vi "DROPBEAR_Model_Updating_Store_Statisitics.vi"(8 "error in (no error)":errorcluster, 11 "DROPBEAR_Model_Updating in":refnum<class "DROPBEAR_Model_Updating.lvclass">) -> (0 "error out":errorcluster, 3 "DROPBEAR_Model_Updating out":refnum<class "DROPBEAR_Model_Updating.lvclass">)   [LabVIEW 2021, in "DROPBEAR_Model_Updating.lvclass"]
uses:
  DROPBEAR_Model_Updating.lvclass
  DROPBEAR_Model_Updating.lvclass/DROPBEAR_Model_Updating.ctl
  Online_Statistic/Online_Statistic.lvclass/Online_Statistic.ctl
  Read Record Statistics.vi
  Write Time Cycle End.vi
  Read Distributional Statistics.vi
  Read Time Flags.vi
  Online_Statistic/Read Cumulative_mean.vi
  Write Distributional Statistics.vi
  Read Online Cycle Time Cost.vi
  Read Time Cycle Start.vi
  Read Time Cycle End.vi
  Write Online Cycle Time Cost.vi
  Read Record Moving Window Data.vi
  Read Record Time Series Data.vi
  Read Pinned State KF.vi
  Read Record Online Error Metrics .vi
  Read Online_SNR_Frequency.vi
  Read Online_SNR_Position_Meters.vi
  Read Online_TRAC_Frequency.vi
  Read Online_TRAC_Meters.vi
  Read Model_Error_Frequency.vi
  Read Model_Error_Meters.vi
  Write Online_SNR_Frequency.vi
  Write Online_SNR_Position_Meters.vi
  Write Online_TRAC_Frequency.vi
  Write Online_TRAC_Meters.vi
  Write Model_Error_Frequency.vi
  Write Model_Error_Meters.vi
  Read Store Statistics Time Cost.vi
  Write Time Store Satistics.vi
  Write Store Statistics Time Cost.vi
  Online_Statistic/Online_Statistic.lvclass
  Moving_Statistic/Moving_Statistic.lvclass
  Data_Array/Data_Array.lvclass
  Kalman_Filter/Kalman_Filter.lvclass
  Online_SNR/Online_SNR.lvclass
  Online_TRAC/Online_TRAC.lvclass
  MOCKBEAR/MOCKBEAR.lvclass
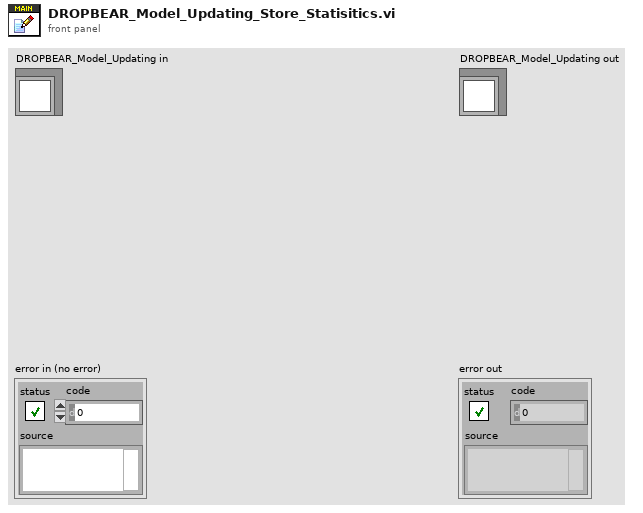
[diagram p1: front panel]
types:
  T1 = cluster{"Data Acquistion Time Cost":refnum<class "Online_Statistic.lvclass">, "FFT Time Cost":refnum<class "Online_Statistic.lvclass">, "Frequency Tracking Time Cost":refnum<class "Online_Statistic.lvclass">, "Sample Location Time Cost":refnum<class "Online_Statistic.lvclass">, "FEA Time Cost":refnum<class "Online_Statistic.lvclass">, "State Tracking Time Cost":refnum<class "Online_Statistic.lvclass">, "Online Cycle Time Cost":refnum<class "Online_Statistic.lvclass">, "Store Statistics Time Cost":refnum<class "Online_Statistic.lvclass">}
  T2 = cluster{"Time Cycle Start":u32, "Time Data Acquire":u32, "Time FFT":u32, "Time KF FFT":u32, "Time Sample":u32, "Time FEA":u32, "Time KF FEA":u32, "Time Cycle End":u32, "Time Store Satistics":u32}
  T3 = cluster{"Displacement Measured Meters":refnum<class "Moving_Statistic.lvclass">, "Displacement Estimate Meters":refnum<class "Moving_Statistic.lvclass">, "Frequency Measured":refnum<class "Moving_Statistic.lvclass">, "Frequency at Estimate":refnum<class "Moving_Statistic.lvclass">}
  T4 = cluster{"Position Measured Meters":dbl, "Position Measured Nodal":i32, "Position Estimated Meters":dbl, "Position Estimated Nodal":i32, "Frequency Estimated KF":dbl, "Frequency Measured FFT":dbl, "Position Estimated Meters KF":dbl, "Position Estimated Nodal KF":i32, "Mean Cycle time":dbl, "Frequency True Position":dbl}
  T5 = cluster{"Modeling Parameters input controls":cluster{"beam_length":dbl, "youngs_modulus":dbl, "torsion_spring":dbl, "beam_height":dbl, "beam_width":dbl, "beam_density":dbl, "number_of_FEA_nodes":i32, "accelerometer_mass":dbl}, "Mockbear input controls":cluster{"Dataset":string, "Resample Method":enum16{"Recorded", "Auto Resample", "Custom Resample"}}, "Simulation Parameters input controls":cluster{"Eigensolver ":enum16{"LabVIEW Cholesky", "LabVIEW General", "LabVIEW Inverse", "LEMP"}, "Models Forcasted":i32, "Max Roller Velocity":dbl, "Max Roller Position Percent":dbl, "Min Roller Position Percent":dbl}, "Program Controls":cluster{"Frequency KF":bool, "Pinned State KF":bool, "FFT Bounding":bool, "Filter Constants Frequency":cluster{"Measurement Variance":dbl, "State Variance":dbl, "Threshold":dbl}, "Filter Constants Position":cluster{"Measurement Variance":dbl, "State Variance":dbl, "Threshold":dbl}, "Moving Window Size":i32, "Time Series buffer":dbl, "Record Time Series Data":bool, "Record Moving Window Data":bool, "Record Online Error Metrics ":bool, "Record Statistics":bool}}
  T6 = cluster{"Frequency KF":bool, "Pinned State KF":bool, "FFT Bounding":bool, "Filter Constants Frequency":cluster{"Measurement Variance":dbl, "State Variance":dbl, "Threshold":dbl}, "Filter Constants Position":cluster{"Measurement Variance":dbl, "State Variance":dbl, "Threshold":dbl}, "Moving Window Size":i32, "Time Series buffer":dbl, "Record Time Series Data":bool, "Record Moving Window Data":bool, "Record Online Error Metrics ":bool, "Record Statistics":bool}
  T7 = cluster{"Displacement Measured Nodal ":refnum<class "Data_Array.lvclass">, "Displacement Measured Meters":refnum<class "Data_Array.lvclass">, "Displacement Estimate Nodal":refnum<class "Data_Array.lvclass">, "Displacement Estimate Meters":refnum<class "Data_Array.lvclass">, "Frequency Measured":refnum<class "Data_Array.lvclass">, "Frequency at Estimate":refnum<class "Data_Array.lvclass">}
  T8 = cluster{"Frequency State":refnum<class "Kalman_Filter.lvclass">, "Rolling Condition State":refnum<class "Kalman_Filter.lvclass">, "Frequency State":dbl, "Pinned Condition State":dbl}
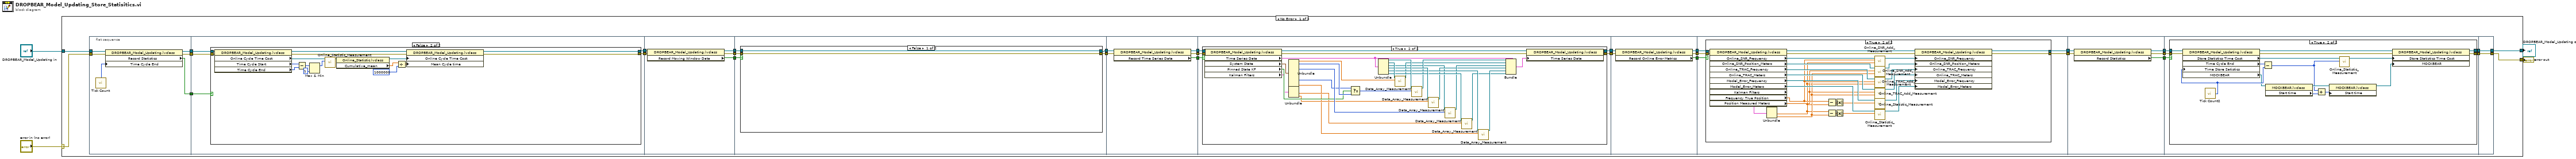
[diagram p0: block diagram]
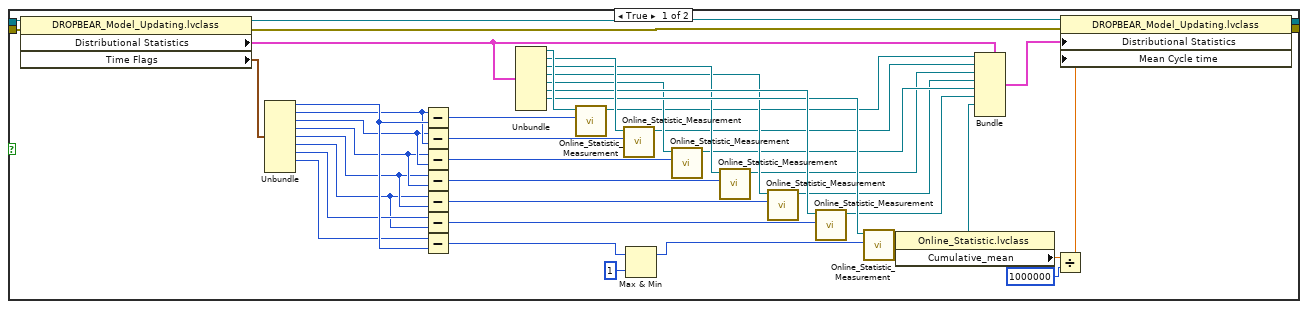
[diagram p2: hidden frame]
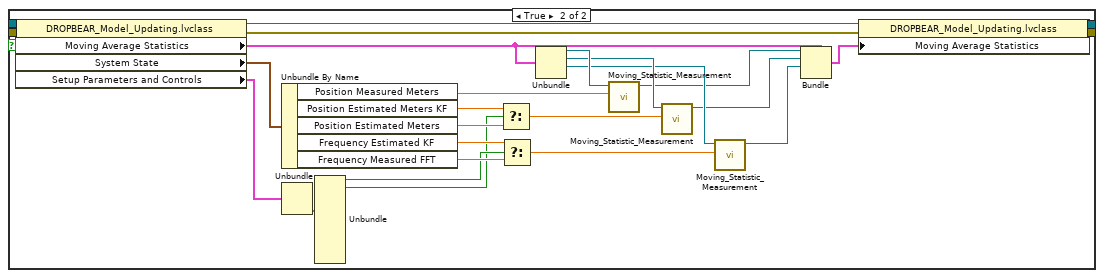
[diagram p3: hidden frame]
diagram:
  n1 = case shown="No Error" "error in (no error)" {
    selector: "error in (no error)" -> [w31 w257]
    tunnel: [w12 w257] -> w3
    tunnel: [w32 w256] -> w1
    tunnel: "DROPBEAR_Model_Updating in" -> [w33 w256]
    frame No Error {
      n2 = flat-sequence {
        tunnel: w31 -> [w38]
        tunnel: w33 -> [w39]
        tunnel: [w37] -> w22
        tunnel: [w36] -> w21
        tunnel: [w35] -> w18
        tunnel: [w44] -> w24
        tunnel: [w43] -> w26
        tunnel: w21 -> [w41]
        tunnel: w22 -> [w42]
        tunnel: w18 -> [w40]
        tunnel: w26 -> [w109]
        tunnel: [w107] -> w25
        tunnel: w24 -> [w110]
        tunnel: [w108] -> w23
        tunnel: [w106] -> w17
        tunnel: [w115] -> w28
        tunnel: [w114] -> w30
        tunnel: w25 -> [w112]
        tunnel: w23 -> [w113]
        tunnel: w17 -> [w111]
        tunnel: w30 -> [w147]
        tunnel: [w145] -> w29
        tunnel: w28 -> [w148]
        tunnel: [w146] -> w27
        tunnel: [w144] -> w16
        tunnel: w29 -> [w150]
        tunnel: w27 -> [w151]
        tunnel: [w153] -> w20
        tunnel: [w152] -> w19
        tunnel: w16 -> [w149]
        tunnel: w20 -> [w191]
        tunnel: w19 -> [w190]
        tunnel: [w189] -> w15
        tunnel: [w188] -> w14
        tunnel: [w187] -> w13
        tunnel: w15 -> [w196]
        tunnel: w14 -> [w195]
        tunnel: w13 -> [w192]
        tunnel: [w194] -> w9
        tunnel: [w193] -> w7
        tunnel: w9 -> [w230]
        tunnel: [w228] -> w8
        tunnel: w7 -> [w229]
        tunnel: [w227] -> w6
        tunnel: [w226] -> w5
        tunnel: w8 -> [w235]
        tunnel: w6 -> [w234]
        tunnel: [w233] -> w11
        tunnel: [w232] -> w10
        tunnel: w5 -> [w231]
        tunnel: [w254] -> w12
        tunnel: [w255] -> w32
        tunnel: w11 -> [w255]
        tunnel: w10 -> [w254]
        frame #0 {
          n3 = call "Tick Count"() -> ("Tick Count(uSec)"=w34:u32)
          n4 = property class="DROPBEAR_Model_Updating.lvclass"(reference=w39, error in=w38, "Time Cycle End"=w34) -> (reference out=w37:refnum<class "DROPBEAR_Model_Updating.lvclass">, error out=w36:errorcluster, "Record Statistics"=w35:bool)
        }
        frame #1 {
          n5 = case shown="False" w40 {
            tunnel: [w66 w104] -> w44
            tunnel: [w64 w102] -> w43
            tunnel: w42 -> [w61 w99]
            tunnel: w41 -> [w51 w98]
            frame True {
              n6 = property class="DROPBEAR_Model_Updating.lvclass"(reference=w61, error in=w51) -> (reference out=w68:refnum<class "DROPBEAR_Model_Updating.lvclass">, error out=w65:errorcluster, "Distributional Statistics"=w75:T1, "Time Flags"=w60:T2)
              n7 = Unbundle(w60) -> ("Time Cycle Start"=w59:u32, "Time Data Acquire"=w56:u32, "Time FFT"=w55:u32, "Time KF FFT"=w54:u32, "Time Sample"=w53:u32, "Time FEA"=w52:u32, "Time KF FEA"=w58:u32, "Time Cycle End"=w57:u32)  [unwired: 1 out]
              n8 = Subtract(x=w56, y=w59) -> (x-y=w88:u32)
              n9 = Subtract(x=w55, y=w56) -> (x-y=w87:u32)
              n10 = Subtract(x=w54, y=w55) -> (x-y=w86:u32)
              n11 = Subtract(x=w53, y=w54) -> (x-y=w85:u32)
              n12 = Subtract(x=w52, y=w53) -> (x-y=w84:u32)
              n13 = Subtract(x=w58, y=w52) -> (x-y=w83:u32)
              n14 = Subtract(x=w57, y=w59) -> (x-y=w47:u32)
              n15 = Unbundle(w75) -> ("Data Acquistion Time Cost"=w82:refnum<class "Online_Statistic.lvclass">, "FFT Time Cost"=w81:refnum<class "Online_Statistic.lvclass">, "Frequency Tracking Time Cost"=w77:refnum<class "Online_Statistic.lvclass">, "Sample Location Time Cost"=w76:refnum<class "Online_Statistic.lvclass">, "FEA Time Cost"=w78:refnum<class "Online_Statistic.lvclass">, "State Tracking Time Cost"=w80:refnum<class "Online_Statistic.lvclass">, "Online Cycle Time Cost"=w79:refnum<class "Online_Statistic.lvclass">)  [unwired: 1 out]
              n16 = call-dynamic "Online_Statistic_Measurement.vi"("New_Measurement"=w88, "Online_Statistic in"=w82) -> ("Online_Statistic out"=w74:refnum<class "Online_Statistic.lvclass">)  [unwired: 8 in, 1 out]
              n17 = call-dynamic "Online_Statistic_Measurement.vi"("New_Measurement"=w87, "Online_Statistic in"=w81) -> ("Online_Statistic out"=w73:refnum<class "Online_Statistic.lvclass">)  [unwired: 8 in, 1 out]
              n18 = Max & Min(x=w47, y=u32 1) -> (max(x,y)=w46:u32)  [unwired: 1 out]
              n19 = call-dynamic "Online_Statistic_Measurement.vi"("New_Measurement"=w86, "Online_Statistic in"=w78) -> ("Online_Statistic out"=w72:refnum<class "Online_Statistic.lvclass">)  [unwired: 8 in, 1 out]
              n20 = call-dynamic "Online_Statistic_Measurement.vi"("New_Measurement"=w85, "Online_Statistic in"=w77) -> ("Online_Statistic out"=w71:refnum<class "Online_Statistic.lvclass">)  [unwired: 8 in, 1 out]
              n21 = call-dynamic "Online_Statistic_Measurement.vi"("New_Measurement"=w84, "Online_Statistic in"=w76) -> ("Online_Statistic out"=w70:refnum<class "Online_Statistic.lvclass">)  [unwired: 8 in, 1 out]
              n22 = call-dynamic "Online_Statistic_Measurement.vi"("New_Measurement"=w83, "Online_Statistic in"=w80) -> ("Online_Statistic out"=w69:refnum<class "Online_Statistic.lvclass">)  [unwired: 8 in, 1 out]
              n23 = call-dynamic "Online_Statistic_Measurement.vi"("New_Measurement"=w46, "Online_Statistic in"=w79) -> ("Online_Statistic out"=w50:refnum<class "Online_Statistic.lvclass">)  [unwired: 8 in, 1 out]
              n24 = property class="Online_Statistic.lvclass"(reference=w50) -> (reference out=w49:refnum<class "Online_Statistic.lvclass">, "Cumulative_mean"=w48:dbl)  [unwired: 1 in, 1 out]
              n25 = Bundle(cluster=w75, "Data Acquistion Time Cost"=w74, "FFT Time Cost"=w73, "Frequency Tracking Time Cost"=w71, "Sample Location Time Cost"=w70, "FEA Time Cost"=w72, "State Tracking Time Cost"=w69, "Online Cycle Time Cost"=w49) -> (w67:T1)  [unwired: 1 in]
              n26 = Divide(x=w48, y=u32 1000000) -> (x/y=w62:dbl)
              n27 = property class="DROPBEAR_Model_Updating.lvclass"(reference=w68, error in=w65, "Distributional Statistics"=w67, "Mean Cycle time"=w62) -> (reference out=w66:refnum<class "DROPBEAR_Model_Updating.lvclass">, error out=w64:errorcluster)
            }
            frame False {
              n28 = property class="DROPBEAR_Model_Updating.lvclass"(reference=w99, error in=w98) -> (reference out=w105:refnum<class "DROPBEAR_Model_Updating.lvclass">, error out=w103:errorcluster, "Online Cycle Time Cost"=w95:refnum<class "Online_Statistic.lvclass">, "Time Cycle Start"=w93:u32, "Time Cycle End"=w92:u32)
              n29 = Subtract(x=w93, y=w92) -> (x-y=w90:u32)
              n30 = Max & Min(x=w90, y=1) -> (max(x,y)=w89:u32)  [unwired: 1 out]
              n31 = call-dynamic "Online_Statistic_Measurement.vi"("New_Measurement"=w89, "Online_Statistic in"=w95) -> ("Online_Statistic out"=w97:refnum<class "Online_Statistic.lvclass">)  [unwired: 8 in, 1 out]
              n32 = property class="Online_Statistic.lvclass"(reference=w97) -> (reference out=w94:refnum<class "Online_Statistic.lvclass">, "Cumulative_mean"=w96:dbl)  [unwired: 1 in, 1 out]
              n33 = Divide(x=w96, y=u32 1000000) -> (x/y=w100:dbl)
              n34 = property class="DROPBEAR_Model_Updating.lvclass"(reference=w105, error in=w103, "Online Cycle Time Cost"=w94, "Mean Cycle time"=w100) -> (reference out=w104:refnum<class "DROPBEAR_Model_Updating.lvclass">, error out=w102:errorcluster)
            }
          }
        }
        frame #2 {
          n35 = property class="DROPBEAR_Model_Updating.lvclass"(reference=w110, error in=w109) -> (reference out=w108:refnum<class "DROPBEAR_Model_Updating.lvclass">, error out=w107:errorcluster, "Record Moving Window Data"=w106:bool)
        }
        frame #3 {
          n36 = case shown="False" w111 {
            tunnel: [w117 w130] -> w115
            tunnel: [w116 w129] -> w114
            tunnel: w113 -> [w117 w128]
            tunnel: w112 -> [w116 w127]
            frame False {
            }
            frame True {
              n37 = property class="DROPBEAR_Model_Updating.lvclass"(reference=w128, error in=w127) -> (reference out=w133:refnum<class "DROPBEAR_Model_Updating.lvclass">, error out=w132:errorcluster, "Moving Average Statistics"=w137:T3, "System State"=w126:T4, "Setup Parameters and Controls"=w125:T5)
              n38 = Unbundle By Name(w126) -> ("Position Measured Meters"=w140:dbl, "Position Estimated Meters KF"=w123:dbl, "Position Estimated Meters"=w122:dbl, "Frequency Estimated KF"=w121:dbl, "Frequency Measured FFT"=w120:dbl)
              n39 = Unbundle(w125) -> ("Program Controls"=w124:T6)  [unwired: 3 out]
              n40 = Unbundle(w124) -> ("Frequency KF"=w119:bool, "Pinned State KF"=w118:bool)  [unwired: 9 out]
              n41 = Select(t=w123, s=w118, f=w122) -> (s? t:f=w139:dbl)
              n42 = Select(t=w121, s=w119, f=w120) -> (s? t:f=w138:dbl)
              n43 = Unbundle(w137) -> ("Displacement Measured Meters"=w143:refnum<class "Moving_Statistic.lvclass">, "Displacement Estimate Meters"=w142:refnum<class "Moving_Statistic.lvclass">, "Frequency Measured"=w141:refnum<class "Moving_Statistic.lvclass">)  [unwired: 1 out]
              n44 = call-dynamic "Moving_Statistic_Measurement.vi"("New_Measurement"=w140, "Moving_Mean in"=w143) -> ("Moving_Mean out"=w136:refnum<class "Moving_Statistic.lvclass">)  [unwired: 8 in, 1 out]
              n45 = call-dynamic "Moving_Statistic_Measurement.vi"("New_Measurement"=w139, "Moving_Mean in"=w142) -> ("Moving_Mean out"=w135:refnum<class "Moving_Statistic.lvclass">)  [unwired: 8 in, 1 out]
              n46 = call-dynamic "Moving_Statistic_Measurement.vi"("New_Measurement"=w138, "Moving_Mean in"=w141) -> ("Moving_Mean out"=w134:refnum<class "Moving_Statistic.lvclass">)  [unwired: 8 in, 1 out]
              n47 = Bundle(cluster=w137, "Displacement Measured Meters"=w136, "Displacement Estimate Meters"=w135, "Frequency Measured"=w134) -> (w131:T3)  [unwired: 1 in]
              n48 = property class="DROPBEAR_Model_Updating.lvclass"(reference=w133, error in=w132, "Moving Average Statistics"=w131) -> (reference out=w130:refnum<class "DROPBEAR_Model_Updating.lvclass">, error out=w129:errorcluster)
            }
          }
        }
        frame #4 {
          n49 = property class="DROPBEAR_Model_Updating.lvclass"(reference=w148, error in=w147) -> (reference out=w146:refnum<class "DROPBEAR_Model_Updating.lvclass">, error out=w145:errorcluster, "Record Time Series Data"=w144:bool)
        }
        frame #5 {
          n50 = case shown="True" w149 {
            tunnel: [w155 w167] -> w153
            tunnel: [w154 w166] -> w152
            tunnel: w151 -> [w155 w165]
            tunnel: w150 -> [w154 w164]
            frame False {
            }
            frame True {
              n51 = property class="DROPBEAR_Model_Updating.lvclass"(reference=w165, error in=w164) -> (reference out=w177:refnum<class "DROPBEAR_Model_Updating.lvclass">, error out=w176:errorcluster, "Time Series Data"=w186:T7, "System State"=w163:T4, "Pinned State KF"=w160:bool, "Kalman Filters"=w159:T8)
              n52 = Unbundle(w163) -> ("Position Measured Meters"=w185:dbl, "Position Measured Nodal"=w162:i32, "Position Estimated Nodal"=w180:i32, "Position Estimated Nodal KF"=w161:i32, "Frequency True Position"=w156:dbl)  [unwired: 5 out]
              n53 = Unbundle(w159) -> ("Frequency State"=w157:dbl, "Pinned Condition State"=w158:dbl)  [unwired: 2 out]
              n54 = Select(t=w161, s=w160, f=w162) -> (s? t:f=w182:i32)
              n55 = Unbundle(w186) -> ("Displacement Measured Nodal"=w183:refnum<class "Data_Array.lvclass">, "Displacement Measured Meters"=w184:refnum<class "Data_Array.lvclass">, "Displacement Estimate Nodal"=w168:refnum<class "Data_Array.lvclass">, "Displacement Estimate Meters"=w181:refnum<class "Data_Array.lvclass">, "Frequency Measured"=w179:refnum<class "Data_Array.lvclass">, "Frequency at Estimate"=w178:refnum<class "Data_Array.lvclass">)
              n56 = call-dynamic "Data_Array_Measurement.vi"("Measurement"=w185, "Data_Array in"=w184) -> ("Data_Array out"=w169:refnum<class "Data_Array.lvclass">)  [unwired: 8 in, 1 out]
              n57 = call-dynamic "Data_Array_Measurement.vi"("Measurement"=w182, "Data_Array in"=w183) -> ("Data_Array out"=w170:refnum<class "Data_Array.lvclass">)  [unwired: 8 in, 1 out]
              n58 = call-dynamic "Data_Array_Measurement.vi"("Measurement"=w158, "Data_Array in"=w181) -> ("Data_Array out"=w171:refnum<class "Data_Array.lvclass">)  [unwired: 8 in, 1 out]
              n59 = call-dynamic "Data_Array_Measurement.vi"("Measurement"=w180, "Data_Array in"=w168) -> ("Data_Array out"=w172:refnum<class "Data_Array.lvclass">)  [unwired: 8 in, 1 out]
              n60 = call-dynamic "Data_Array_Measurement.vi"("Measurement"=w157, "Data_Array in"=w178) -> ("Data_Array out"=w173:refnum<class "Data_Array.lvclass">)  [unwired: 8 in, 1 out]
              n61 = call-dynamic "Data_Array_Measurement.vi"("Measurement"=w156, "Data_Array in"=w179) -> ("Data_Array out"=w174:refnum<class "Data_Array.lvclass">)  [unwired: 8 in, 1 out]
              n62 = Bundle(cluster=w186, "Displacement Measured Nodal"=w170, "Displacement Measured Meters"=w169, "Displacement Estimate Nodal"=w172, "Displacement Estimate Meters"=w171, "Frequency Measured"=w174, "Frequency at Estimate"=w173) -> (w175:T7)
              n63 = property class="DROPBEAR_Model_Updating.lvclass"(reference=w177, error in=w176, "Time Series Data"=w175) -> (reference out=w167:refnum<class "DROPBEAR_Model_Updating.lvclass">, error out=w166:errorcluster)
            }
          }
        }
        frame #6 {
          n64 = property class="DROPBEAR_Model_Updating.lvclass"(reference=w191, error in=w190) -> (reference out=w189:refnum<class "DROPBEAR_Model_Updating.lvclass">, error out=w188:errorcluster, "Record Online Error Metrics "=w187:bool)
        }
        frame #7 {
          n65 = case shown="True" w192 {
            tunnel: w196 -> [w198 w225]
            tunnel: w195 -> [w197 w224]
            tunnel: [w198 w211] -> w194
            tunnel: [w197 w210] -> w193
            frame False {
            }
            frame True {
              n66 = property class="DROPBEAR_Model_Updating.lvclass"(reference=w225, error in=w224) -> (reference out=w213:refnum<class "DROPBEAR_Model_Updating.lvclass">, error out=w212:errorcluster, "Online_SNR_Frequency"=w223:refnum<class "Online_SNR.lvclass">, "Online_SNR_Position_Meters"=w222:refnum<class "Online_SNR.lvclass">, "Online_TRAC_Frequency"=w221:refnum<class "Online_TRAC.lvclass">, "Online_TRAC_Meters"=w220:refnum<class "Online_TRAC.lvclass">, "Model_Error_Frequency"=w219:refnum<class "Online_Statistic.lvclass">, "Model_Error_Meters"=w218:refnum<class "Online_Statistic.lvclass">, "Kalman Filters"=w203:T8, "Frequency True Position"=w202:dbl, "Position Measured Meters"=w201:dbl)
              n67 = Unbundle(w203) -> ("Frequency State"=w199:dbl, "Pinned Condition State"=w200:dbl)  [unwired: 2 out]
              n68 = Subtract(x=w202, y=w199) -> (x-y=w217:dbl)
              n69 = Subtract(x=w199, y=w200) -> (x-y=w216:dbl)
              n70 = Absolute Value(x=w217) -> (abs(x)=w214:dbl)
              n71 = Absolute Value(x=w216) -> (abs(x)=w215:dbl)
              n72 = call-dynamic "Online_SNR_Add_Measurement.vi"("Estimate"=w199, "True"=w202, "Online_SNR in"=w223) -> ("Online_SNR out"=w209:refnum<class "Online_SNR.lvclass">)  [unwired: 7 in, 1 out]
              n73 = call-dynamic "Online_SNR_Add_Measurement.vi"("Estimate"=w200, "True"=w201, "Online_SNR in"=w222) -> ("Online_SNR out"=w208:refnum<class "Online_SNR.lvclass">)  [unwired: 7 in, 1 out]
              n74 = call-dynamic "Online_TRAC_Add_Measurement.vi"("Estimate"=w199, "True"=w202, "Online_TRAC in"=w221) -> ("Online_TRAC out"=w207:refnum<class "Online_TRAC.lvclass">)  [unwired: 7 in, 1 out]
              n75 = call-dynamic "Online_TRAC_Add_Measurement.vi"("Estimate"=w200, "True"=w201, "Online_TRAC in"=w220) -> ("Online_TRAC out"=w206:refnum<class "Online_TRAC.lvclass">)  [unwired: 7 in, 1 out]
              n76 = call-dynamic "Online_Statistic_Measurement.vi"("New_Measurement"=w214, "Online_Statistic in"=w219) -> ("Online_Statistic out"=w205:refnum<class "Online_Statistic.lvclass">)  [unwired: 8 in, 1 out]
              n77 = call-dynamic "Online_Statistic_Measurement.vi"("New_Measurement"=w215, "Online_Statistic in"=w218) -> ("Online_Statistic out"=w204:refnum<class "Online_Statistic.lvclass">)  [unwired: 8 in, 1 out]
              n78 = property class="DROPBEAR_Model_Updating.lvclass"(reference=w213, error in=w212, "Online_SNR_Frequency"=w209, "Online_SNR_Position_Meters"=w208, "Online_TRAC_Frequency"=w207, "Online_TRAC_Meters"=w206, "Model_Error_Frequency"=w205, "Model_Error_Meters"=w204) -> (reference out=w211:refnum<class "DROPBEAR_Model_Updating.lvclass">, error out=w210:errorcluster)
            }
          }
        }
        frame #8 {
          n79 = property class="DROPBEAR_Model_Updating.lvclass"(reference=w230, error in=w229) -> (reference out=w228:refnum<class "DROPBEAR_Model_Updating.lvclass">, error out=w227:errorcluster, "Record Statistics"=w226:bool)
        }
        frame #9 {
          n80 = case shown="True" w231 {
            tunnel: w235 -> [w237 w253]
            tunnel: w234 -> [w236 w252]
            tunnel: [w237 w245] -> w233
            tunnel: [w236 w244] -> w232
            frame False {
            }
            frame True {
              n81 = call "Tick Count2"() -> ("Tick Count(uSec)"=w250:u32)
              n82 = property class="DROPBEAR_Model_Updating.lvclass"(reference=w253, error in=w252, "Time Store Satistics"=w250) -> (reference out=w248:refnum<class "DROPBEAR_Model_Updating.lvclass">, error out=w246:errorcluster, "Store Statistics Time Cost"=w249:refnum<class "Online_Statistic.lvclass">, "Time Cycle End"=w251:u32, "MOCKBEAR"=w243:refnum<class "MOCKBEAR.lvclass">)
              n83 = Subtract(x=w251, y=w250) -> (x-y=w238:u32)
              n84 = property class="MOCKBEAR.lvclass"(reference=w243) -> (reference out=w242:refnum<class "MOCKBEAR.lvclass">, "Start time"=w239:u32)  [unwired: 1 in, 1 out]
              n85 = Add(x=w238, y=w239) -> (x+y=w240:u32)
              n86 = property class="MOCKBEAR.lvclass"(reference=w242, "Start time"=w240) -> (reference out=w241:refnum<class "MOCKBEAR.lvclass">)  [unwired: 1 in, 1 out]
              n87 = call-dynamic "Online_Statistic_Measurement.vi"("New_Measurement"=w238, "Online_Statistic in"=w249) -> ("Online_Statistic out"=w247:refnum<class "Online_Statistic.lvclass">)  [unwired: 8 in, 1 out]
              n88 = property class="DROPBEAR_Model_Updating.lvclass"(reference=w248, error in=w246, "Store Statistics Time Cost"=w247, "MOCKBEAR"=w241) -> (reference out=w245:refnum<class "DROPBEAR_Model_Updating.lvclass">, error out=w244:errorcluster)
            }
          }
        }
        frame #10 {
        }
      }
    }
    frame Error {
    }
  }
  "error out" <- w3
  "DROPBEAR_Model_Updating out" <- w1
